vi "Test panel positioning.vi"() -> ()   [LabVIEW 2012]
uses:
  <vilib>/Utility/miscctls.llb/LVRectTypeDef.ctl
  <vilib>/Utility/miscctls.llb/LVBoundsTypeDef.ctl
  <vilib>/Utility/miscctls.llb/LVPositionTypeDef.ctl
panel:
  out "FP Pos":T1
  out "FP Bounds":T2
  out "output cluster":T1
  out "Bounds":T2
  out "Front Panel Window:Window Bounds":T3
  out "SWIPE!!!":bool
  in  "OK Button":bool
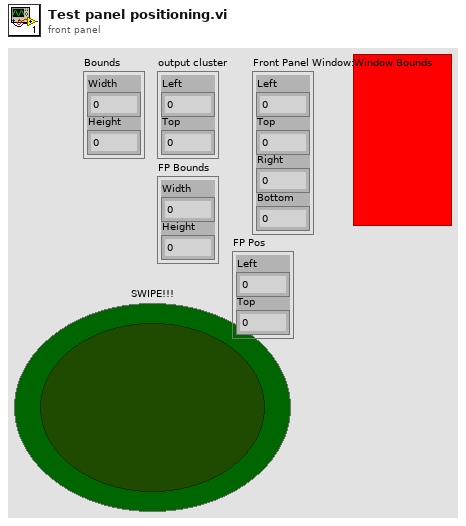
[diagram p1: front panel]
types:
  T1 = typedef "LVPositionTypeDef.ctl" = cluster{"Left":i32, "Top":i32}
  T2 = typedef "LVBoundsTypeDef.ctl" = cluster{"Width":u32, "Height":u32}
  T3 = typedef "LVRectTypeDef.ctl" = cluster{"Left":i16, "Top":i16, "Right":i16, "Bottom":i16}
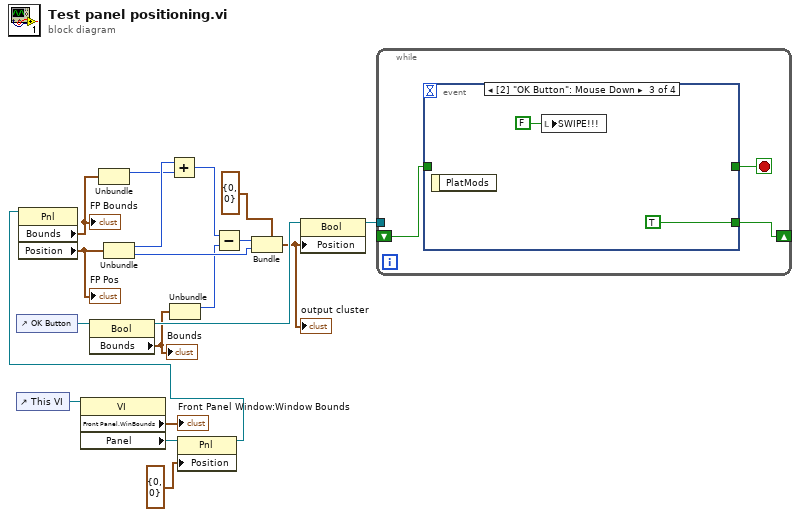
[diagram p0: block diagram]
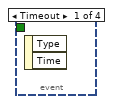
[diagram p2: hidden frame]
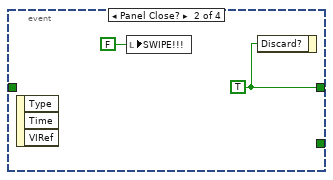
[diagram p3: hidden frame]
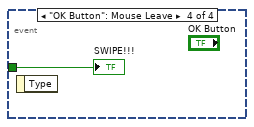
[diagram p4: hidden frame]
diagram:
  n1 = control-ref of="OK Button"() -> (w18:refnum<vi>)
  n2 = control-ref of="This VI"() -> (w4:refnum<vi>)
  n3 = property class="VI"(reference=w4) -> ("Front Panel.WinBounds"=→"Front Panel Window:Window Bounds":T3, "Panel"=w3:refnum<vi>)  [unwired: 1 in, 2 out]
  n4 = property class="Bool"(reference=w18) -> (reference out=w17:refnum<vi>, "Bounds"=w16:T2)  [unwired: 1 in, 1 out]
  "Bounds" <- w16
  n5 = Unbundle(w16) -> ("Width"=w6:u32)  [unwired: 1 out]
  n6 = property class="Pnl"(reference=w3, "Position"=T1 {"Left"=0, "Top"=0}) -> (reference out=w1:refnum<vi>)  [unwired: 1 in, 1 out]
  n7 = property class="Pnl"(reference=w1) -> ("Bounds"=w9:T2, "Position"=w12:T1)  [unwired: 1 in, 2 out]
  "FP Bounds" <- w9
  "FP Pos" <- w12
  n8 = Unbundle(w9) -> ("Width"=w8:u32)  [unwired: 1 out]
  n9 = Unbundle(w12) -> ("Left"=w10:i32, "Top"=w11:i32)
  n10 = Add(x=w10, y=w8) -> (x+y=w7:u32)
  n11 = Subtract(x=w7, y=w6) -> (x-y=w5:u32)
  n12 = Bundle(cluster=T1 {"Left"=0, "Top"=0} ("Position"), "Left"=w5, "Top"=w11) -> (w15:T1)
  "output cluster" <- w15
  n13 = property class="Bool"(reference=w17, "Position"=w15) -> (reference out=w13:refnum<vi>)  [unwired: 1 in, 1 out]
  n14 = while {
    shift-right: [w21] -> _
    shift-left: _ -> [w20]
    tunnel: w13 -> [_]
    stop <- w22 stop-if-true
    n15 = event shown="[2] \"OK Button\": Mouse Down" {
      selector: _ -> [_ _ _ _]
      dyn-events: _ -> [_ _ _ _]
      timeout: _ -> [_ _ _ _]
      tunnel: [_ w24 _ _] -> w22
      tunnel: [_ _ TRUE _] -> w21
      tunnel: w20 -> [_ _ _ w27]
      event Timeout {
        n16 = event-data() -> ()  [unwired: 1 in, 2 out]
      }
      event Panel Close? {
        w24 = TRUE ("Discard?")
        n17 = event-data() -> ()  [unwired: 1 in, 3 out]
        n18 = local write "SWIPE!!!"(FALSE ("SWIPE!!!")) -> ()
        n19 = event-data("Discard?"=w24) -> ()  [unwired: 1 in, 1 out]
      }
      event "OK Button": Mouse Down {
        n20 = event-data() -> ()  [unwired: 1 in, 1 out]
        n21 = local write "SWIPE!!!"(FALSE ("SWIPE!!!")) -> ()
      }
      event "OK Button": Mouse Leave {
        n22 = event-data() -> ()  [unwired: 1 in, 1 out]
        "SWIPE!!!" <- w27
      }
    }
  }
